vi "Escape VI Name.vi"(11 "Path":string) -> (3 "Escaped":string)   [LabVIEW 2015, in "CLI.lvclass"]
uses:
  CLI.lvclass
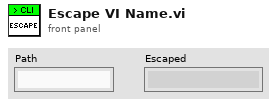
[diagram p1: front panel]
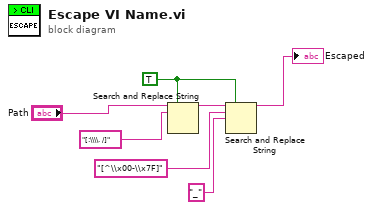
[diagram p0: block diagram]
diagram:
  w5 = TRUE ("replace all? (F)")
  n1 = Search and Replace String(replace all?=w5, input string="Path", search string="[:\\\\. /]") -> (result string=w3:string)  [unwired: 5 in, 3 out]
  n2 = Search and Replace String(replace all?=w5, input string=w3, search string="[^\\x00-\\x7F]", replace string="_" ("replace string (\"\")")) -> (result string=→"Escaped":string)  [unwired: 4 in, 3 out]
